vi "Create All Message Queues.vi"(8 "error in (no error)":errorcluster) -> (0 "error out":errorcluster, 3 "Message Queues out":T1)   [LabVIEW 2015, in "Message Queue.lvlib"]
doc: "This VI creates and initializes all the message queues for your application. If your application requires more than one message queue, right-click the \"Message Queues\" constant above and select Open Type Def. Add the new Message Queue(s) to the type definition, then initialize them in this VI."
uses:
  Message Queue.lvlib
  Message Cluster.ctl
  All Message Queues.ctl
  Enqueue Message (Single).vi
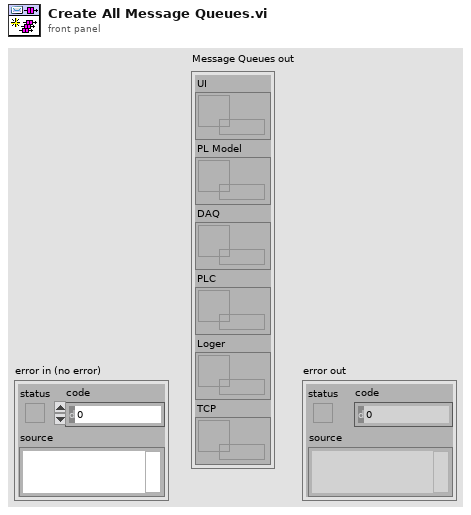
[diagram p1: front panel]
types:
  T1 = typedef "Message Queue.lvlib/All Message Queues.ctl" = cluster{"UI":refnum<queue>, "PL Model":refnum<queue>, "DAQ":refnum<queue>, "PLC":refnum<queue>, "Loger":refnum<queue>, "TCP":refnum<queue>}
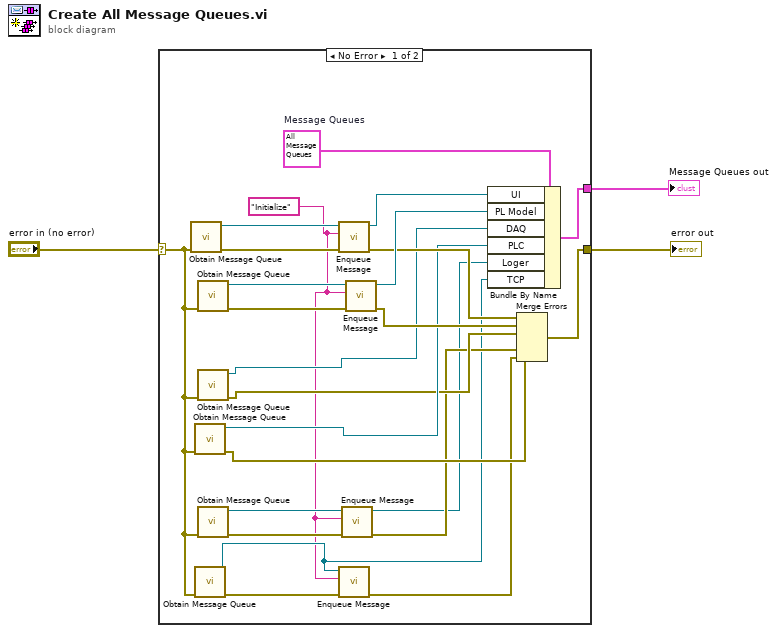
[diagram p0: block diagram]
diagram:
  n1 = case shown="No Error" "error in (no error)" {
    selector: "error in (no error)" -> [w8 w28]
    tunnel: [w17 w28] -> w3
    tunnel: [w26 _] -> w2
    frame No Error {
      w4 = "Initialize" ("Message")
      w27 = T1 {"UI"=refnum, "PL Model"=refnum, "DAQ"=refnum, "PLC"=refnum, "Loger"=refnum, "TCP"=refnum}  # Message Queues
      n2 = call "Obtain Message Queue.vi"("error in (no error)"=w8) -> ("error out"=w25:errorcluster, "Message Queue"=w24:refnum<queue>)  [unwired: 9 in]
      n3 = call "Obtain Message Queue.vi"("error in (no error)"=w8) -> ("error out"=w13:errorcluster, "Message Queue"=w15:refnum<queue>)  [unwired: 9 in]
      n4 = call "Obtain Message Queue.vi"("error in (no error)"=w8) -> ("error out"=w7:errorcluster, "Message Queue"=w5:refnum<queue>)  [unwired: 9 in]
      n5 = call "Obtain Message Queue.vi"("error in (no error)"=w8) -> ("error out"=w22:errorcluster, "Message Queue"=w23:refnum<queue>)  [unwired: 9 in]
      n6 = call "Obtain Message Queue.vi"("error in (no error)"=w8) -> ("error out"=w14:errorcluster, "Message Queue"=w16:refnum<queue>)  [unwired: 9 in]
      n7 = call "Obtain Message Queue.vi"("error in (no error)"=w8) -> ("error out"=w12:errorcluster, "Message Queue"=w11:refnum<queue>)  [unwired: 9 in]
      n8 = call-poly "Enqueue Message.vi"("error in (no error)"=w25, "Message"=w4, "Message Queue"=w24) -> ("error out"=w19:errorcluster, "dup Message Queue"=w20:refnum<queue>)  [unwired: 7 in]
      n9 = call-poly "Enqueue Message.vi"("error in (no error)"=w7, "Message"=w4, "Message Queue"=w5) -> ("error out"=w6:errorcluster)  [unwired: 7 in, 1 out]
      n10 = call-poly "Enqueue Message.vi"("error in (no error)"=w12, "Message"=w4, "Message Queue"=w11) -> ("error out"=w10:errorcluster, "dup Message Queue"=w9:refnum<queue>)  [unwired: 7 in]
      n11 = call-poly "Enqueue Message.vi"("error in (no error)"=w22, "Message"=w4, "Message Queue"=w23) -> ("error out"=w18:errorcluster, "dup Message Queue"=w21:refnum<queue>)  [unwired: 7 in]
      n12 = Bundle By Name(cluster=w27, "UI"=w20, "PL Model"=w21, "DAQ"=w16, "PLC"=w15, "Loger"=w9, "TCP"=w5) -> (w26:T1)
      n13 = Merge Errors(w19, w18, w14, w13, w10, w6) -> (w17:errorcluster)
    }
    frame Error {
    }
  }
  "Message Queues out" <- w2
  "error out" <- w3
